vi "record_signal.vi"(6 "onoff":bool=TRUE, 7 "file_base_name":string="signal", 9 "value_array":dbl[](array[numeric]), 11 "date_time":timestamp) -> ()   [LabVIEW 2019]
uses:
  <vilib>/Utility/file.llb/Write Delimited Spreadsheet (string).vi
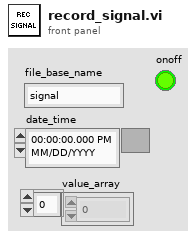
[diagram p1: front panel]
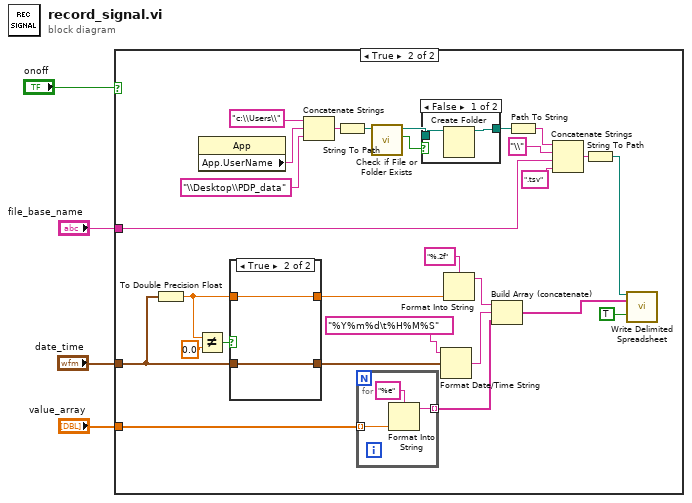
[diagram p0: block diagram]
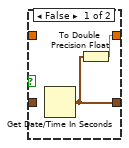
[diagram p3: hidden frame]
diagram:
  n1 = case shown="True" "onoff" {
    tunnel: "file_base_name" -> [_ w25]
    tunnel: "date_time" -> [_ w14]
    tunnel: "value_array" -> [_ w5]
    frame False {
    }
    frame True {
      n2 = To Double Precision Float(number=w14) -> (double precision float=w10:dbl)
      n3 = Not Equal?(x=w10, y=0.0) -> (x != y?=w16:bool)
      n4 = property class="App"() -> ("App.UserName"=w29:string)  [unwired: 2 in, 2 out]
      n5 = case shown="True" w16 {
        tunnel: [w36 w39] -> w7
        tunnel: w14 -> [_ w39]
        tunnel: [w37 w38] -> w11
        tunnel: w10 -> [_ w38]
        frame False {
          n6 = Get Date/Time In Seconds() -> (seconds since 1Jan1904=w36:timestamp)
          n7 = To Double Precision Float(number=w36) -> (double precision float=w37:dbl)
        }
        frame True {
        }
      }
      n8 = Concatenate Strings("c:\\Users\\", w29, "\\Desktop\\PDP_data") -> (w27:string)
      n9 = String To Path(string=w27) -> (path=w22:path)
      n10 = for {
        tunnel: [w35] -> w12 mode=indexing
        tunnel: w5 -> [w34] mode=indexing
        n11 = Format Into String(format string="%e", w34) -> (resulting string=w35:string)  [unwired: 2 in, 1 out]
      }
      n12 = call <vilib>:"Check if File or Folder Exists.vi"("path"=w22) -> ("file or folder exists?"=w21:bool, "dup path"=w19:path)  [unwired: 8 in, 1 out]
      n13 = case shown="False" w21 {
        tunnel: w19 -> [w41 w42]
        tunnel: [w40 w42] -> w20
        frame False {
          n14 = Create Folder(path (use dialog)=w41) -> (created path=w40:path)  [unwired: 2 in, 2 out]
        }
        frame True {
        }
      }
      n15 = Format Date/Time String(time format string (%c)="%Y%m%d\t%H%M%S" ("format string"), seconds (now)=w7) -> (date/time string=w8:string)  [unwired: 1 in]
      n16 = Format Into String(format string="%.2f", w11) -> (resulting string=w13:string)  [unwired: 2 in, 1 out]
      n17 = Build Array (concatenate)(w13, w8, w12) -> (w32:string[])
      n18 = Path To String(path=w20) -> (string=w18:string)
      n19 = Concatenate Strings(w18, "\\", w25, ".tsv" ("string")) -> (w23:string)
      n20 = String To Path(string=w23) -> (path=w17:path)
      n21 = call-poly <vilib>:"Write Delimited Spreadsheet.vi"("file path (dialog if empty)"=w17, "1D data"=w32, "append to file? (new file:F)"=TRUE) -> ()  [unwired: 11 in, 2 out]
    }
  }
